vi "Get Axis No Objects.vi"(8 "error in (no error)":errorcluster, 11 "Synapse CCD in":T1={"JYCCDLib.IJYCCDReqd"=refnum, "JYMONOLib.IJYMonoReqd"=refnum, "Integration time"=0.01, "ADC"=0, "GAIN"=0, "areas :"=[[1, 1, 1, 1024, 256, 1, 256]], "Most Recent Data Object"=refnum, "Mono Properties"={"Grating"=0, "Center Wavelength"=0.0, "Entrance Slit"=0.0, "Exit Slit"=0.0}, "Coverage"={"Max"=0.0, "Min"=0.0}, "Multi-Acquisitions"={"Dark Subtract?"=FALSE, "Averaging?"=FALSE, "Cosmic Ray Removal?"=FALSE, "# to Average"=0, "Time Between Acq."=0, "Acquisitions Control Array"=[TRUE], "Raw Data"=[], "Processed Data"=[], "Array of Wavelengths"=[]}, "Channel Names"=["Wavelength", "Signal"], "Channel Units"=["nm", "counts"]} {"ADC" items=["   20 kHz", "1 MHz", "1 MHz Ultra"]; "GAIN" items=["High Light", "Best Dynamic", "High Sensitivity"]; "Mono Properties"."Grating" items=["1200 lines/mm - 500 nm Blaze", "1200 lines/mm - 750 nm Blaze", "600 lines/mm - 1000 nm Blaze"]}) -> (0 "error out":errorcluster, 2 "Array of Wavelengths":dbl[](array[numeric]), 3 "Synapse CCD out":T1={"JYCCDLib.IJYCCDReqd"=refnum, "JYMONOLib.IJYMonoReqd"=refnum, "Integration time"=0.01, "ADC"=0, "GAIN"=0, "areas :"=[[1, 1, 1, 1024, 256, 1, 256]], "Most Recent Data Object"=refnum, "Mono Properties"={"Grating"=0, "Center Wavelength"=0.0, "Entrance Slit"=0.0, "Exit Slit"=0.0}, "Coverage"={"Max"=0.0, "Min"=0.0}, "Multi-Acquisitions"={"Dark Subtract?"=FALSE, "Averaging?"=FALSE, "Cosmic Ray Removal?"=FALSE, "# to Average"=0, "Time Between Acq."=0, "Acquisitions Control Array"=[TRUE], "Raw Data"=[], "Processed Data"=[], "Array of Wavelengths"=[]}, "Channel Names"=["Wavelength", "Signal"], "Channel Units"=["nm", "counts"]} {"ADC" items=["   20 kHz", "1 MHz", "1 MHz Ultra"]; "GAIN" items=["High Light", "Best Dynamic", "High Sensitivity"]; "Mono Properties"."Grating" items=["1200 lines/mm - 500 nm Blaze", "1200 lines/mm - 750 nm Blaze", "600 lines/mm - 1000 nm Blaze"]})   [LabVIEW 2009]
doc: "Reads the linearized wavelengths from last Data Acquisition, returns as Array of DBLs."
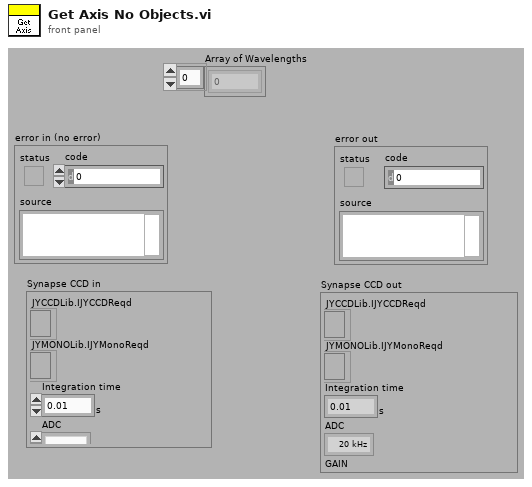
[diagram p1: front panel]
types:
  T1 = cluster{"JYCCDLib.IJYCCDReqd":refnum<k7>, "JYMONOLib.IJYMonoReqd":refnum<k7>, "Integration time":dbl[unit], "ADC":u16, "GAIN":u16, "areas :":i32[][], "Most Recent Data Object":refnum<k7>, "Mono Properties":cluster{"Grating":u16, "Center Wavelength":dbl[unit], "Entrance Slit":dbl[unit], "Exit Slit":dbl[unit]}, "Coverage":cluster{"Max":dbl[unit], "Min":dbl[unit]}, "Multi-Acquisitions":cluster{"Dark Subtract?":bool, "Averaging?":bool, "Cosmic Ray Removal?":bool, "# to Average":u32, "Time Between Acq.":u32, "Acquisitions Control Array":bool[], "Raw Data":i32[][], "Processed Data":dbl[], "Array of Wavelengths":dbl[]}, "Channel Names":string[], "Channel Units":string[]}
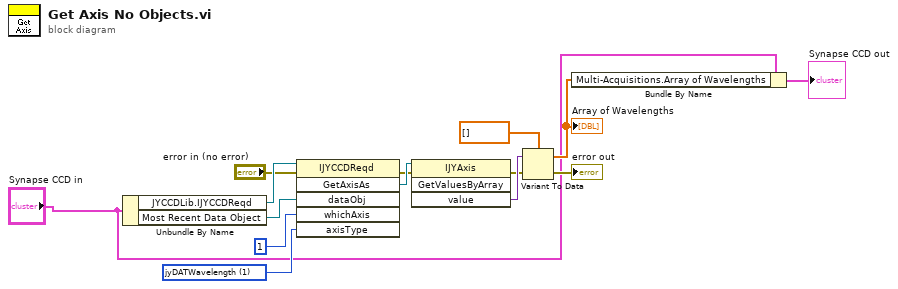
[diagram p0: block diagram]
diagram:
  w12 = 1 items=["jyDATUndefined", "jyDATWavelength", "jyDATPixel", "jyDATMillimeters", "jyDATMicrometers"] ("axisType")
  n1 = Unbundle By Name("Synapse CCD in") -> ("JYCCDLib.IJYCCDReqd"=w14:refnum<k7>, "Most Recent Data Object"=w13:refnum<k7>)
  n2 = invoke class="IJYCCDReqd" method="GetAxisAs"(reference=w14, error in="error in (no error)", "dataObj"=w13, "whichAxis"=1, "axisType"=w12) -> (error out=w9:errorcluster, "GetAxisAs"=w10:refnum<k7>)  [unwired: 1 in, 4 out]
  n3 = invoke class="IJYAxis" method="GetValuesByArray"(reference=w10, error in=w9) -> (error out=w6:errorcluster, "value"=w8:variant)  [unwired: 2 in, 2 out]
  n4 = Variant To Data(error in=w6, Variant=w8, type=dbl[] []) -> (error out=→"error out":errorcluster, data=w3:dbl[])
  "Array of Wavelengths" <- w3
  n5 = Bundle By Name(cluster="Synapse CCD in", "Multi-Acquisitions.Array of Wavelengths"=w3) -> (→"Synapse CCD out":T1)
